vi "Open_xlsx.vi"(2 "错误输入（无错误）":errorcluster, 3 "excel路径":path, 4 "document引用":refnum<k7>) -> (0 "错误输出":errorcluster, 1 "该文档引用输出":refnum<k7>)   [LabVIEW 2014]
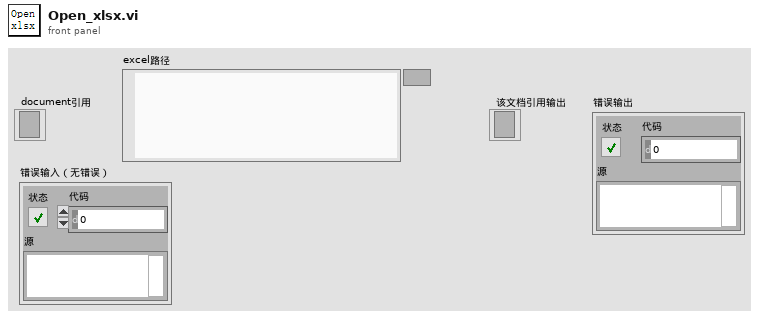
[diagram p1: front panel]
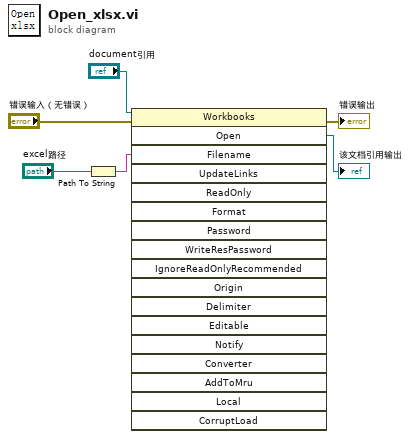
[diagram p0: block diagram]
diagram:
  n1 = Path To String(path="excel路径") -> (string=w5:string)
  n2 = invoke class="Workbooks" method="Open"(reference="document引用", error in="错误输入（无错误）", "Filename"=w5) -> (error out=→"错误输出":errorcluster, "Open"=→"该文档引用输出":refnum<k7>)  [unwired: 15 in, 16 out]
